vi "Configure Transform Function.vi"(8 "error in (no error)":errorcluster, 9 "Transform Function (0: Time)":i32(ring) items=["Time", "Distance"], 10 "Channel (1)":i32=1, 11 "VISA resource name":refnum<visa-resource-name>) -> (0 "error out":errorcluster, 3 "VISA resource name out":refnum<visa-resource-name>)   [LabVIEW 2020, in "Agilent ENA Series.lvlib"]
doc: "Specifies the transform function.\n\n<B>Note:</B>This VI is only valid on E5061B."
uses:
  <instrlib>/Agilent ENA Series/Agilent ENA Series.lvlib
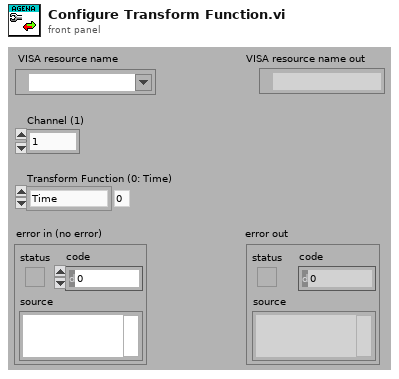
[diagram p1: front panel]
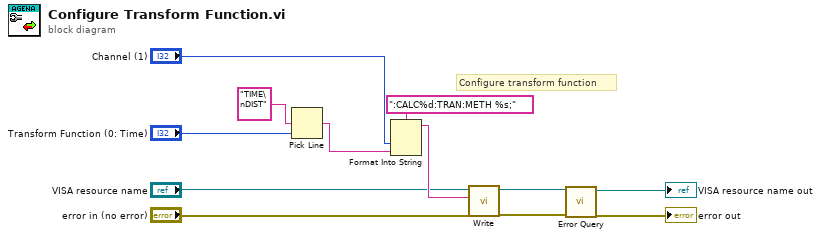
[diagram p0: block diagram]
diagram:
  # "Configure transform function"
  n1 = Pick Line(multi-line string="TIME\nDIST", line index="Transform Function (0: Time)") -> (output string=w8:string)  [unwired: 1 out]
  n2 = Format Into String(format string=":CALC%d:TRAN:METH %s;", "Channel (1)", w8) -> (resulting string=w3:string)  [unwired: 2 in, 1 out]
  n3 = call <instrlib>:"Write.vi"("error in (no error)"="error in (no error)", "String ()"=w3, "VISA resource name"="VISA resource name") -> ("error out"=w4:errorcluster, "VISA resource name out"=w5:refnum<visa-resource-name>)  [unwired: 6 in, 1 out]
  n4 = call <instrlib>:"Error Query.vi"("error in (no error)"=w4, "VISA resource name"=w5) -> ("error out"=→"error out":errorcluster, "VISA resource name out"=→"VISA resource name out":refnum<visa-resource-name>)  [unwired: 8 out]
